vi "2D Array (Normal).vi"(0 "rows":i32=2, 2 "cols":i32=4, 4 "mean":dbl, 5 "std":dbl=1.0, 8 "Fixed Seed":bool=TRUE) -> (15 "Array":dbl[][](array[numeric])=[[0.21505248184279538, 1.4489319414399218, 0.748829957623609, 0.8509848240921414], [1.6209332090971538, -2.2206908717027742, 0.7729092217163482, 1.0927445780488823]] format="%.3f")   [LabVIEW 2014]
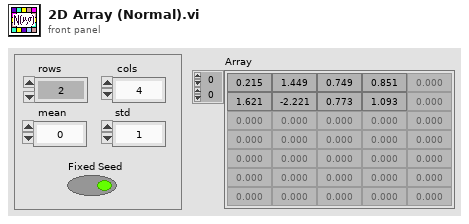
[diagram p1: front panel]
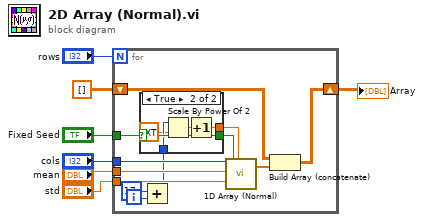
[diagram p0: block diagram]
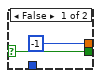
[diagram p2: hidden frame]
diagram:
  n1 = for {
    N: "rows" -> [_]
    tunnel: "cols" -> [w19]
    tunnel: "mean" -> [w18]
    tunnel: "std" -> [w17]
    shift-right: [w15] -> w3
    shift-left: dbl[][] [] -> [w14]
    tunnel: "Fixed Seed" -> [w13]
    i -> [w10]
    n2 = Add(x=17, y=w10) -> (x+y=w9:i32)
    n3 = case shown="True" w13 {
      selector: w13 -> [w20 w26]
      tunnel: [-1 w25] -> w12
      tunnel: [w20 w26] -> w11
      tunnel: w9 -> [_ w23]
      frame False {
      }
      frame True {
        n4 = Scale By Power Of 2(n=w23, x=ext 1.0) -> (x*2^n=w24:ext)
        n5 = Increment(x=w24) -> (x+1=w25:ext)
      }
    }
    n6 = call "1D Array (Normal).vi"("samples"=w19, "mean"=w18, "std"=w17, "fixed seed"=w11, "seed"=w12) -> ("normal random data"=w16:dbl[])  [unwired: 14 in]
    n7 = Build Array (concatenate)(w14, w16) -> (w15:dbl[][])
  }
  "Array" <- w3
